vi "fetch_data.vi"(8 "error in (no error)":errorcluster, 11 "GenericToplevelComponent in":refnum<class "GenericToplevelComponent.lvclass">) -> (0 "error out":errorcluster, 2 "data out":variant, 3 "GenericToplevelComponent out":refnum<class "GenericToplevelComponent.lvclass">, 4 "# elements in queue":i32)   [LabVIEW 2010, in "GenericToplevelComponent.lvclass"]
uses:
  GenericToplevelComponent.lvclass
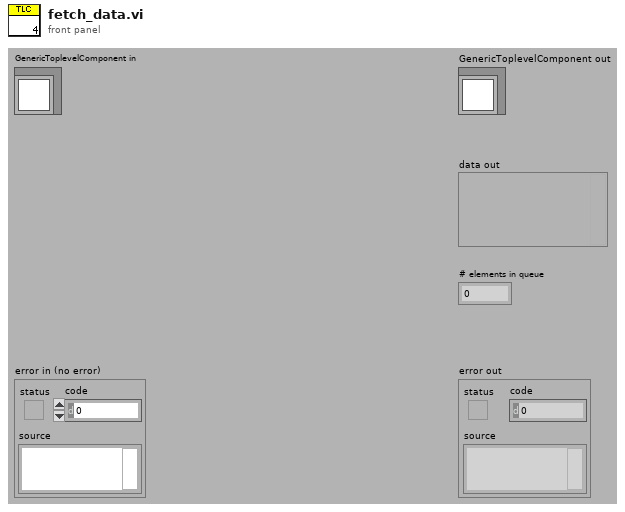
[diagram p1: front panel]
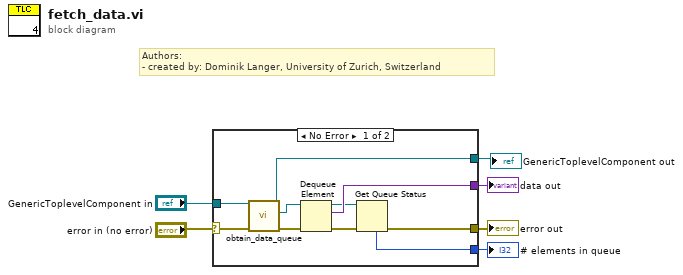
[diagram p0: block diagram]
diagram:
  # "Authors: \n- created by: Dominik Langer, University of Zurich, Switzerland"
  n1 = case shown="No Error" "error in (no error)" {
    selector: "error in (no error)" -> [w16 w18]
    tunnel: [w8 w18] -> w3
    tunnel: [w14 w17] -> w4
    tunnel: "GenericToplevelComponent in" -> [w15 w17]
    tunnel: [w12 _] -> w1
    tunnel: [w10 _] -> w2
    frame No Error {
      n2 = call-dynamic "obtain_data_queue.vi"("error in (no error)"=w16, "GenericToplevelComponent in"=w15) -> ("error out"=w11:errorcluster, "data queue"=w13:refnum<queue>, "GenericToplevelComponent out"=w14:refnum<class "GenericToplevelComponent.lvclass">)  [unwired: 7 in]
      n3 = Dequeue Element(queue=w13, error in (no error)=w11) -> (queue out=w7:refnum<queue>, element=w12:variant, error out=w9:errorcluster)  [unwired: 1 in, 1 out]
      n4 = Get Queue Status(queue=w7, error in (no error)=w9) -> (error out=w8:errorcluster, # elements in queue=w10:i32)  [unwired: 1 in, 6 out]
    }
    frame Error {
    }
  }
  "error out" <- w3
  "GenericToplevelComponent out" <- w4
  "# elements in queue" <- w2
  "data out" <- w1
